vi "Init.vi"(8 "error in (no error)":errorcluster, 11 "Data in":refnum<class "DAQmx - Analog Input Single Sample.lvclass">) -> (0 "error out":errorcluster, 3 "Data out":refnum<class "DAQmx - Analog Input Single Sample.lvclass">)   [LabVIEW 2021, in "DAQmx - Analog Input Single Sample.lvclass"]
doc: "Abstract Data Classes 2.1.1.13\nTim Streeter - TSA\nCopyright (c) 2025, TSA"
uses:
  DAQmx - Analog Input Single Sample.lvclass
  C:/Program Files (x86)/National Instruments/LabVIEW 2021/vi.lib/TSA/Omni-Bus/Omni-Bus/Bus Access/Bus_Access.lvclass
  C:/TSA/DAQmx-Bus/Source/DAQmx-Bus.lvclass
  <vilib>/TSA/Omni-Bus/Omni-Bus/Bus Access/Bus_Access.lvclass/Bus_Access.ctl
  DAQmx - Analog Input Single Sample.lvclass/DAQmx - Analog Input Single Sample.ctl
  Types/DBL/DAQmx-Bus_DBL_Type.lvclass
  C:/Program Files (x86)/National Instruments/LabVIEW 2021/vi.lib/TSA/Abstract Data Classes/Abs_Types/Value/Abs_Value.lvclass
  C:/Program Files (x86)/National Instruments/LabVIEW 2021/vi.lib/TSA/Abstract Data Classes/Abs_Types/Type/Abs_Type.lvclass
  Types/DBL/DAQmx-Bus_DBL_Type.lvclass/DAQmx-Bus_DBL_Type.ctl
  DAQmx-Bus.lvclass/DAQmx-Bus.ctl
  Types/DBL/Properties/Write Values DVR.vi
  Types/DBL/Properties/Write Index.vi
  <vilib>/TSA/Omni-Bus/Omni-Bus/Bus Access/Properties/Read Tags.vi
  Properties/Write Actor Ref.vi
  <vilib>/TSA/Omni-Bus/Omni-Bus/Bus Access/Properties/Write Values.vi
  Support/Actor.vi
  DAQmx-Bus.lvclass
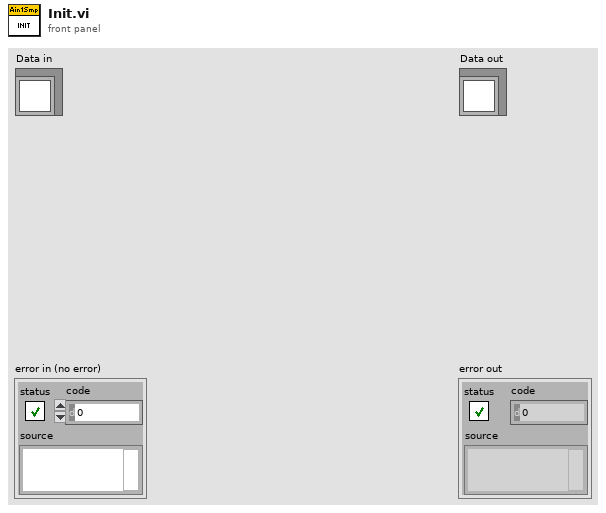
[diagram p1: front panel]
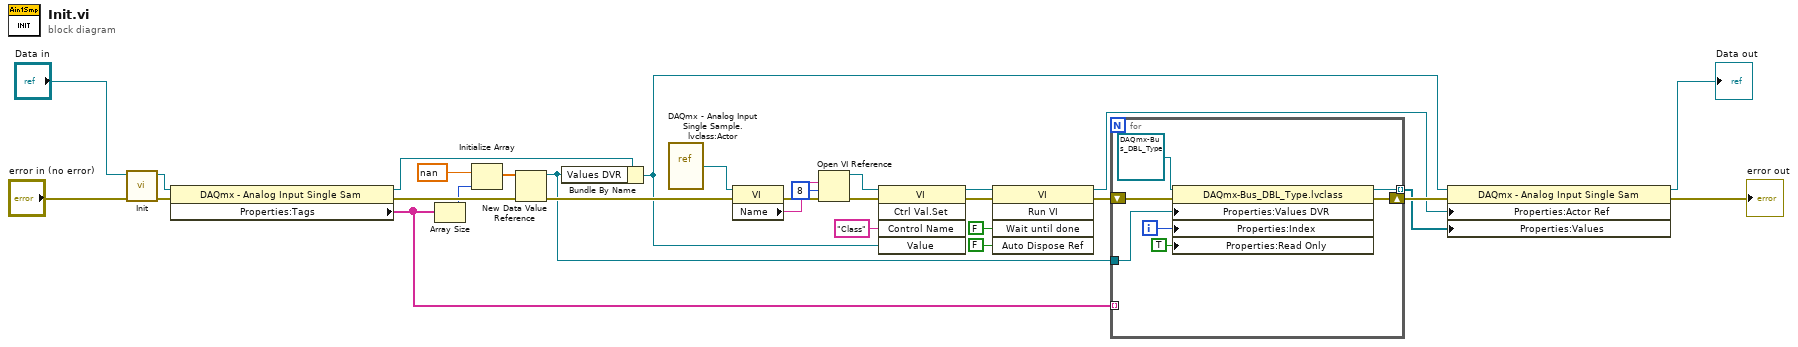
[diagram p0: block diagram]
diagram:
  n1 = call-parent "Init.vi"("error in (no error)"="error in (no error)", "Data in"="Data in") -> ("error out"=w19:errorcluster, "Data out"=w18:refnum<class "DAQmx - Analog Input Single Sample.lvclass">)  [unwired: 8 in]
  n2 = property class="DAQmx - Analog Input Single Sam"(reference=w18, error in=w19) -> (reference out=w13:refnum<class "DAQmx - Analog Input Single Sample.lvclass">, error out=w17:errorcluster, "Properties:Tags"=w11:string[])
  n3 = Array Size(array=w11) -> (size(s)=w16:i32)
  n4 = Initialize Array(nan, w16) -> (w14:dbl[])
  n5 = New Data Value Reference(data value=w14, error in=w17) -> (data value reference=w9:refnum<data-value>, error out=w28:errorcluster)
  n6 = Bundle By Name(cluster=w13, "Values DVR"=w9) -> (w10:refnum<class "DAQmx - Analog Input Single Sample.lvclass">)
  n7 = vi-ref "DAQmx - Analog Input Single Sample.lvclass:Actor.vi"() -> (w27:refnum<vi>)
  n8 = property class="VI"(reference=w27, error in=w28) -> (error out=w25:errorcluster, "Name"=w26:string)  [unwired: 1 out]
  n9 = Open VI Reference(vi path=w26, options=8, error in (no error)=w25) -> (vi reference=w23:refnum<vi>, error out=w24:errorcluster)  [unwired: 3 in]
  n10 = invoke class="VI" method="Ctrl Val.Set"(reference=w23, error in=w24, "Control Name"="Class", "Value"=w10) -> (reference out=w6:refnum<vi>, error out=w5:errorcluster)  [unwired: 1 in, 3 out]
  n11 = invoke class="VI" method="Run VI"(reference=w6, error in=w5, "Wait until done"=FALSE ("Wait Until Done"), "Auto Dispose Ref"=FALSE ("Auto Dispose Reference")) -> (reference out=w3:refnum<vi>, error out=w4:errorcluster)  [unwired: 1 in, 3 out]
  n12 = for {
    shift-right: [w35] -> w12
    shift-left: w4 -> [w36]
    tunnel: w11 -> [_] mode=indexing
    tunnel: w9 -> [w33]
    tunnel: [w32] -> w8 mode=indexing
    i -> [w34]
    n13 = property class="DAQmx-Bus_DBL_Type.lvclass"(reference=refnum<class "DAQmx-Bus_DBL_Type.lvclass"> refnum ("DAQmx-Bus_DBLType.lvclass"), error in=w36, "Properties:Values DVR"=w33, "Properties:Index"=w34, "Properties:Read Only"=TRUE ("Read Only")) -> (reference out=w32:refnum<class "DAQmx-Bus_DBL_Type.lvclass">, error out=w35:errorcluster)
  }
  n14 = property class="DAQmx - Analog Input Single Sam"(reference=w10, error in=w12, "Properties:Actor Ref"=w3, "Properties:Values"=w8) -> (reference out=→"Data out":refnum<class "DAQmx - Analog Input Single Sample.lvclass">, error out=→"error out":errorcluster)
